vi "niScope Create Configuration List Step.vi"(0 "instrument handle":refnum<k15>, 1 "set as active step":bool=TRUE, 11 "error in":errorcluster) -> (4 "instrument handle out":refnum<k15>, 15 "error out":errorcluster)   [LabVIEW 2013]
doc: "Use this function to create a step in a Configuration List that is active. The created step has default values for all the attributes that are in the list. Set the setAsActiveStep parameter to make this step the active one."
uses:
  niScope_32.dll
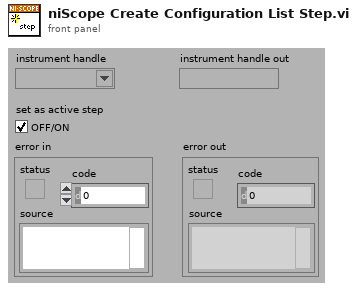
[diagram p1: front panel]
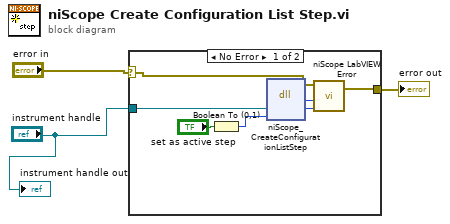
[diagram p0: block diagram]
diagram:
  n1 = case shown="No Error" "error in" {
    selector: "error in" -> [w6 w11]
    tunnel: [w7 w11] -> w2
    tunnel: "instrument handle" -> [w10 _]
    frame No Error {
      n2 = Boolean To (0,1)(Boolean="set as active step") -> (0, 1=w4:i16)
      n3 = dll-call lib="niScope_*.*" fn="niScope_CreateConfigurationListStep" ("niScope_32.*:niScope_CreateConfigurationStep")("instrument handle"=w10, "setAsActiveStep"=w4) -> ("status"=w9:i32, "instrument handle"=w8:u32)  [unwired: 3 in, 3 out]
      n4 = call <instrlib>:"niScope LabVIEW Error.vi"("instrument handle"=w8, "niScope error code (0)"=w9, "error in (no error)"=w6) -> ("error out"=w7:errorcluster)  [unwired: 2 out]
    }
    frame Error {
    }
  }
  "error out" <- w2
  "instrument handle out" <- "instrument handle"
